vi "LoadGlobais.vi"(8 "error in (no error)":errorcluster, 11 "Device in":refnum<class "Device.lvclass">) -> (0 "error out":errorcluster, 2 "Resp":string, 3 "Device out":refnum<class "Device.lvclass">)   [LabVIEW 2012]
uses:
  Device.lvclass
  Global Coude.vi
  <vilib>/Utility/config.llb/NI_LVConfig.lvlib
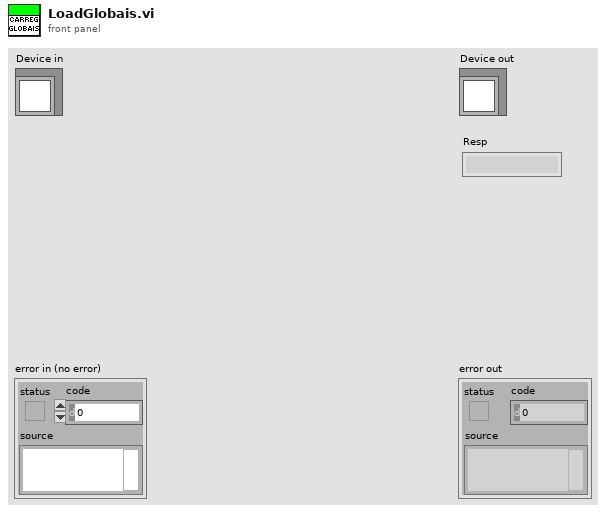
[diagram p1: front panel]
types:
  T1 = cluster{"Mec ID":string, "VISA Mec":refnum<visa-resource-name>, "Mec PosLimit":string, "Mec NegLimit":string, "Mec Factor":dbl, "Mec Speed":dbl, "Mec Acceleration":dbl, "MecOffset":string, "MecTargets":dbl[], "MecEnabled":bool, "Mec Target":dbl}
  T2 = typedef "NI_LVConfig.lvlib/Config Data RefNum.ctl" = refnum<k1>
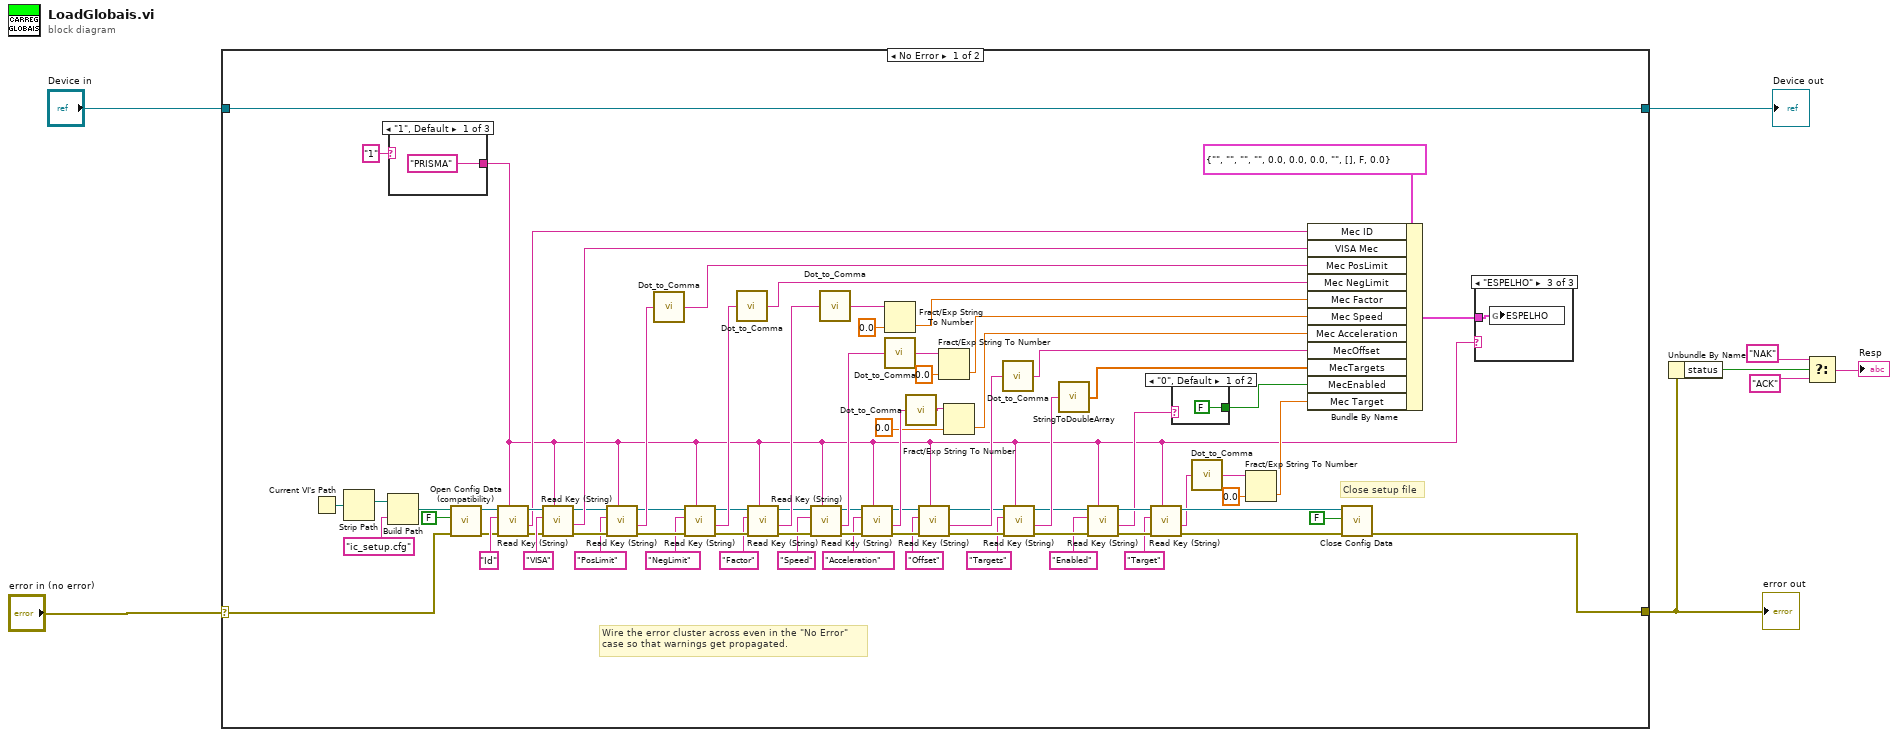
[diagram p0: block diagram]
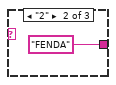
[diagram p2: hidden frame]
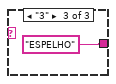
[diagram p3: hidden frame]
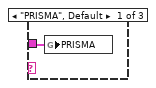
[diagram p4: hidden frame]
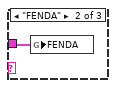
[diagram p5: hidden frame]
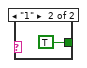
[diagram p6: hidden frame]
diagram:
  n1 = case shown="No Error" "error in (no error)" {
    selector: "error in (no error)" -> [w11 w94]
    tunnel: [w10 w94] -> w1
    tunnel: [w13 w93] -> w6
    tunnel: "Device in" -> [w13 w93]
    frame No Error {
      # "Close setup file"
      # "Wire the error cluster across even in the \"No Error\"\ncase so that warnings get propagated."
      n2 = Current VI's Path() -> (path=w38:path)
      n3 = Strip Path(path=w38) -> (stripped path=w39:path)  [unwired: 1 out]
      n4 = Build Path(base path=w39, name or relative path="ic_setup.cfg") -> (appended path=w19:path)
      n5 = case shown="\"1\", Default" "1" {
        tunnel: ["PRISMA" "FENDA" "ESPELHO"] -> w12
        frame "1", Default {
        }
        frame "2" {
        }
        frame "3" {
        }
      }
      n6 = call <vilib>:"Open Config Data (compatibility).vi"("error in (no error)"=w11, "create file if necessary (T)"=FALSE ("create file if necessary? (T)"), "configuration file path"=w19) -> ("error out"=w17:errorcluster, "refnum"=w16:T2)  [unwired: 6 in, 1 out]
      n7 = call <vilib>:"Read Key (String).vi"("section"=w12, "error in (no error)"=w17, "key"="Id", "refnum"=w16) -> ("error out"=w21:errorcluster, "value"=w20:string, "refnum out"=w22:T2)  [unwired: 2 in, 3 out]
      n8 = call <vilib>:"Read Key (String).vi"("section"=w12, "error in (no error)"=w21, "key"="VISA", "refnum"=w22) -> ("error out"=w63:errorcluster, "value"=w77:string, "refnum out"=w59:T2)  [unwired: 2 in, 3 out]
      n9 = call <vilib>:"Read Key (String).vi"("section"=w12, "error in (no error)"=w63, "key"="PosLimit", "refnum"=w59) -> ("error out"=w65:errorcluster, "value"=w69:string, "refnum out"=w64:T2)  [unwired: 2 in, 3 out]
      n10 = call "Dot_to_Comma.vi"("String in"=w69) -> ("String out"=w78:string)
      n11 = call <vilib>:"Read Key (String).vi"("section"=w12, "error in (no error)"=w65, "key"="NegLimit", "refnum"=w64) -> ("error out"=w62:errorcluster, "value"=w70:string, "refnum out"=w58:T2)  [unwired: 2 in, 3 out]
      n12 = call "Dot_to_Comma.vi"("String in"=w70) -> ("String out"=w79:string)
      n13 = call <vilib>:"Read Key (String).vi"("section"=w12, "error in (no error)"=w62, "key"="Factor", "refnum"=w58) -> ("error out"=w61:errorcluster, "value"=w71:string, "refnum out"=w57:T2)  [unwired: 2 in, 3 out]
      n14 = call <vilib>:"Read Key (String).vi"("section"=w12, "error in (no error)"=w61, "key"="Speed", "refnum"=w57) -> ("error out"=w60:errorcluster, "value"=w67:string, "refnum out"=w56:T2)  [unwired: 2 in, 3 out]
      n15 = call "Dot_to_Comma.vi"("String in"=w71) -> ("String out"=w72:string)
      n16 = call <vilib>:"Read Key (String).vi"("section"=w12, "error in (no error)"=w60, "key"="Acceleration", "refnum"=w56) -> ("error out"=w51:errorcluster, "value"=w73:string, "refnum out"=w50:T2)  [unwired: 2 in, 3 out]
      n17 = Fract/Exp String To Number(string=w72, default (0 dbl)=0.0 ("default (0 DBL)")) -> (number=w80:dbl)  [unwired: 3 out]
      n18 = call "Dot_to_Comma.vi"("String in"=w67) -> ("String out"=w68:string)
      n19 = call "Dot_to_Comma.vi"("String in"=w73) -> ("String out"=w74:string)
      n20 = call <vilib>:"Read Key (String).vi"("section"=w12, "error in (no error)"=w51, "key"="Offset", "refnum"=w50) -> ("error out"=w49:errorcluster, "value"=w75:string, "refnum out"=w48:T2)  [unwired: 2 in, 3 out]
      n21 = Fract/Exp String To Number(string=w68, default (0 dbl)=0.0) -> (number=w81:dbl)  [unwired: 3 out]
      n22 = Fract/Exp String To Number(string=w74, default (0 dbl)=0.0) -> (number=w82:dbl)  [unwired: 3 out]
      n23 = call "Dot_to_Comma.vi"("String in"=w75) -> ("String out"=w83:string)
      n24 = call <vilib>:"Read Key (String).vi"("section"=w12, "error in (no error)"=w49, "key"="Targets", "refnum"=w48) -> ("error out"=w34:errorcluster, "value"=w41:string, "refnum out"=w37:T2)  [unwired: 2 in, 3 out]
      n25 = call "StringToDoubleArray.vi"("String"=w41) -> ("MecTargets"=w84:dbl[])
      n26 = call <vilib>:"Read Key (String).vi"("section"=w12, "error in (no error)"=w34, "key"="Enabled", "refnum"=w37) -> ("error out"=w33:errorcluster, "value"=w29:string, "refnum out"=w36:T2)  [unwired: 2 in, 3 out]
      n27 = call <vilib>:"Read Key (String).vi"("section"=w12, "error in (no error)"=w33, "key"="Target", "refnum"=w36) -> ("error out"=w32:errorcluster, "value"=w25:string, "refnum out"=w35:T2)  [unwired: 2 in, 3 out]
      n28 = case shown="\"0\", Default" w29 {
        tunnel: [FALSE TRUE] -> w28
        frame "0", Default {
        }
        frame "1" {
        }
      }
      n29 = call "Dot_to_Comma.vi"("String in"=w25) -> ("String out"=w27:string)
      n30 = Fract/Exp String To Number(string=w27, default (0 dbl)=0.0) -> (number=w24:dbl)  [unwired: 3 out]
      n31 = Bundle By Name(cluster=T1 {"Mec ID"="", "VISA Mec"="", "Mec PosLimit"="", "Mec NegLimit"="", "Mec Factor"=0.0, "Mec Speed"=0.0, "Mec Acceleration"=0.0, "MecOffset"="", "MecTargets"=[], "MecEnabled"=FALSE, "Mec Target"=0.0} ("CAM"), "Mec ID"=w20, "VISA Mec"=w77, "Mec PosLimit"=w78, "Mec NegLimit"=w79, "Mec Factor"=w80, "Mec Speed"=w81, "Mec Acceleration"=w82, "MecOffset"=w83, "MecTargets"=w84, "MecEnabled"=w28, "Mec Target"=w24) -> (w15:T1)
      n32 = call <vilib>:"Close Config Data.vi"("error in (no error)"=w32, "write file if changed (T)"=FALSE ("create file if necessary? (T)"), "refnum"=w35) -> ("error out"=w10:errorcluster)  [unwired: 8 out]
      n33 = case shown="\"ESPELHO\"" w12 {
        tunnel: w15 -> [w88 w89 w90]
        frame "PRISMA", Default {
          n34 = global write "Global Coude.vi" "PRISMA"(w88) -> ()
        }
        frame "FENDA" {
          n35 = global write "Global Coude.vi" "FENDA"(w89) -> ()
        }
        frame "ESPELHO" {
          n36 = global write "Global Coude.vi" "ESPELHO"(w90) -> ()
        }
      }
    }
    frame Error {
    }
  }
  "error out" <- w1
  "Device out" <- w6
  n37 = Unbundle By Name(w1) -> ("status"=w5:bool)
  n38 = Select(t="NAK", s=w5, f="ACK") -> (s? t:f=→"Resp":string)
